vi "Save Project For Previous Version.vi"(8 "Error In":errorcluster, 9 "LabVIEW Version":T1, 10 "Save Directory":path, 11 "Project Path":path) -> (0 "Error Out":errorcluster, 2 "Warnings":string)   [LabVIEW 2011, in "LVH-Toolbox.lvlib" / "LVH-Common.lvlib"]
uses:
  LVH-Common.lvlib
  Private/Type Defs/LabVIEW Version.ctl
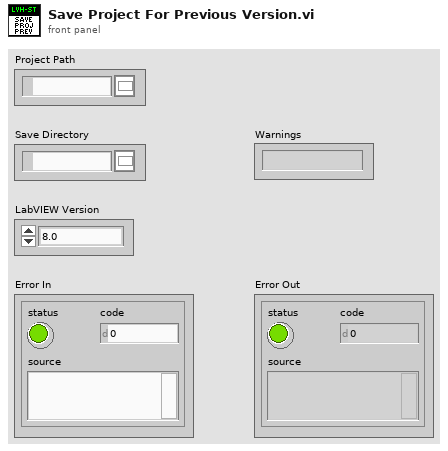
[diagram p1: front panel]
types:
  T1 = typedef "LVH-Toolbox.lvlib/LVH-Common.lvlib/LabVIEW Version.ctl" = enum16{"8.0", "8.2", "8.6", "9.0", "10.0", "11.0", "12.0", "13.0"}
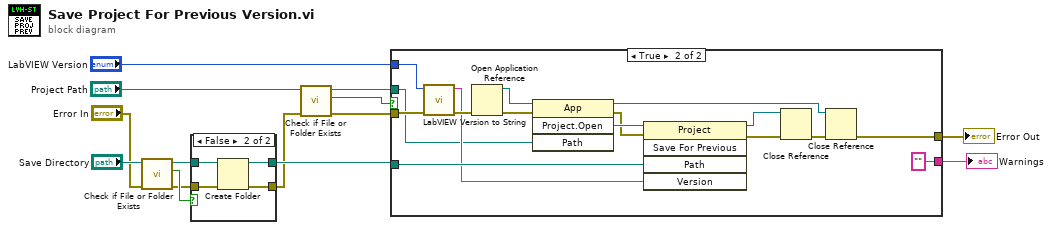
[diagram p0: block diagram]
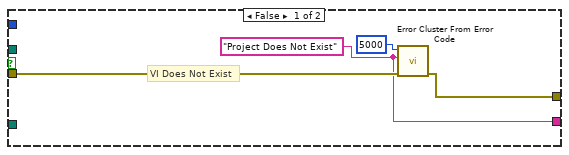
[diagram p3: hidden frame]
diagram:
  n1 = call <vilib>:"Check if File or Folder Exists.vi"("error in (no error)"="Error In", "path"="Save Directory") -> ("error out"=w2:errorcluster, "file or folder exists?"=w3:bool, "dup path"=w5:path)  [unwired: 7 in]
  n2 = case shown="False" w3 {
    tunnel: w5 -> [w16 w20]
    tunnel: [w16 w19] -> w4
    tunnel: w2 -> [w15 w18]
    tunnel: [w15 w17] -> w1
    frame True {
    }
    frame False {
      n3 = Create Folder(path (use dialog)=w20, error in=w18) -> (created path=w19:path, error out=w17:errorcluster)  [unwired: 1 in, 1 out]
    }
  }
  n4 = call <vilib>:"Check if File or Folder Exists.vi"("error in (no error)"=w1, "path"="Project Path") -> ("error out"=w11:errorcluster, "file or folder exists?"=w13:bool, "dup path"=w12:path)  [unwired: 7 in]
  n5 = case shown="True" w13 {
    tunnel: w12 -> [_ w26]
    tunnel: w11 -> [w23 w39]
    tunnel: w4 -> [_ w28]
    tunnel: [w24 w29] -> w10
    tunnel: [w21 "" ("error message (\"\")")] -> w9
    tunnel: "LabVIEW Version" -> [_ w40]
    frame False {
      w21 = "Project Does Not Exist" ("error message (\"\")")
      # "VI Does Not Exist"
      n6 = call <vilib>:"Error Cluster From Error Code.vi"("error in (no error)"=w23, "error message (\"\")"=w21, "error code (0)"=5000) -> ("error out"=w24:errorcluster)  [unwired: 6 in]
    }
    frame True {
      n7 = call "LabVIEW Version to String.vi"("Error In"=w39, "LabVIEW Version"=w40) -> ("Error Out"=w30:errorcluster, "LabVIEW Version"=w27:string)  [unwired: 8 in]
      n8 = Open Application Reference(8:w30) -> (0:w38:errorcluster, 3:w37:refnum<vi>)  [unwired: 3 in]
      n9 = invoke class="App" method="Project.Open"(reference=w37, error in=w38, "Path"=w26) -> (reference out=w31:refnum<vi>, error out=w35:errorcluster, "Project:Open"=w36:refnum<vi>)  [unwired: 1 in, 1 out]
      n10 = invoke class="Project" method="Save For Previous"(reference=w36, error in=w35, "Path"=w28, "Version"=w27) -> (reference out=w33:refnum<vi>, error out=w34:errorcluster)  [unwired: 1 in, 3 out]
      n11 = Close Reference(reference=w33, error in (no error)=w34) -> (error out=w32:errorcluster)
      n12 = Close Reference(reference=w31, error in (no error)=w32) -> (error out=w29:errorcluster)
    }
  }
  "Error Out" <- w10
  "Warnings" <- w9
